vi "Y_AxisMotorControlSetupAndHome.vi"() -> ()   [LabVIEW 2020]
uses:
  C:/Program Files/National Instruments/LabVIEW 2020/examples/Instrument IO/Serial/support/Serial - Settings.ctl
  <vilib>/Instr/_visa.llb/VISA Configure Serial Port (Instr).vi
panel:
  out "read buffer 2":string
  out "read buffer 3":string
  out "7":bool
  out "6":bool
  out "5":bool
  out "4":bool
  out "3":bool
  out "8":bool
  out "2":bool
  out "1":bool
  in  "Serial Com Port":refnum<visa-resource-name>="COM3"
  out "read buffer":string
  in  "Serial Settings":T1={"baud rate"=57600, "data bits"=8, "parity"=enum."None", "stop bits"=10, "flow control"=0} {"flow control" items=["None"=0, "XON/XOFF"=1, "RTS/CTS"=2, "DTR/DSR"=4]; "stop bits" items=["1.0"=10, "1.5"=15, "2.0"=20]; "data bits" min=5 max=8 step=1; "baud rate" items=["75"=75, "110"=110, "134"=134, "150"=150, "300"=300, "600"=600, "1200"=1200, "1800"=1800, "2400"=2400, "4800"=4800, "7200"=7200, "9600"=9600, "14400"=14400, "19200"=19200, "28800"=28800, "38400"=38400, "56000"=56000, "57600"=57600, "115200"=115200, "128000"=128000, "230400"=230400]}
  out "Status Array":bool[](array[boolean])
  out "Limit Switch Status":i32 format="%b"
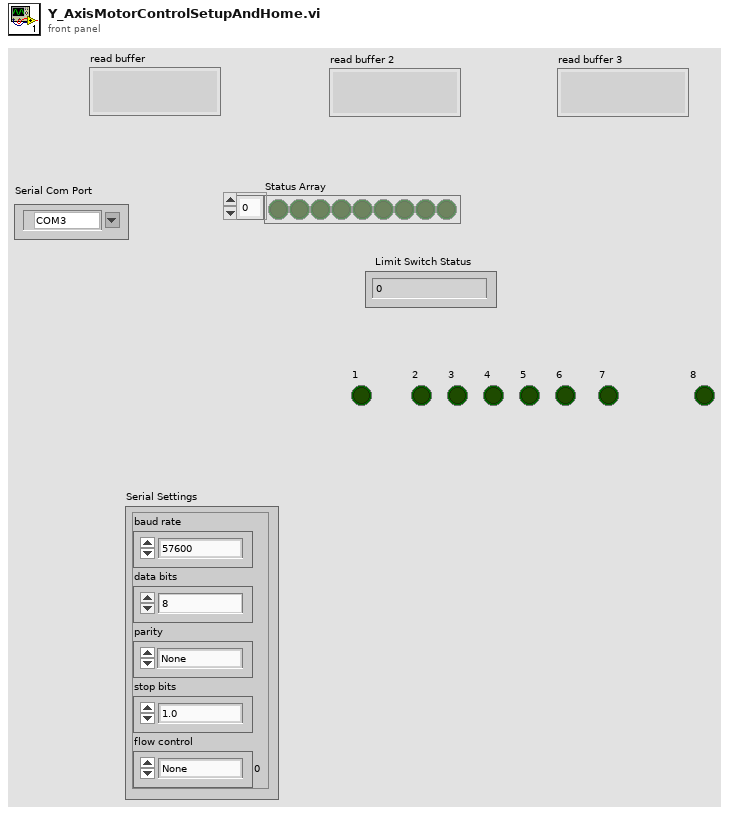
[diagram p1: front panel]
types:
  T1 = typedef "Serial - Settings.ctl" = cluster{"baud rate":u32, "data bits":u16, "parity":enum16{"None", "Odd", "Even", "Mark", "Space"}, "stop bits":u16, "flow control":u16}
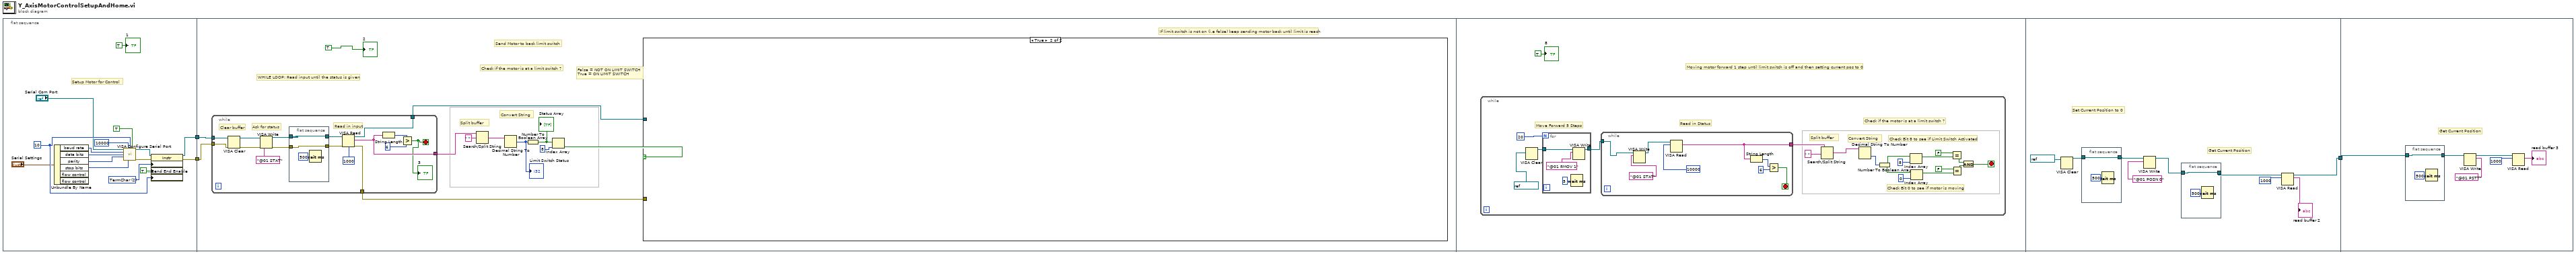
[diagram p0: block diagram]
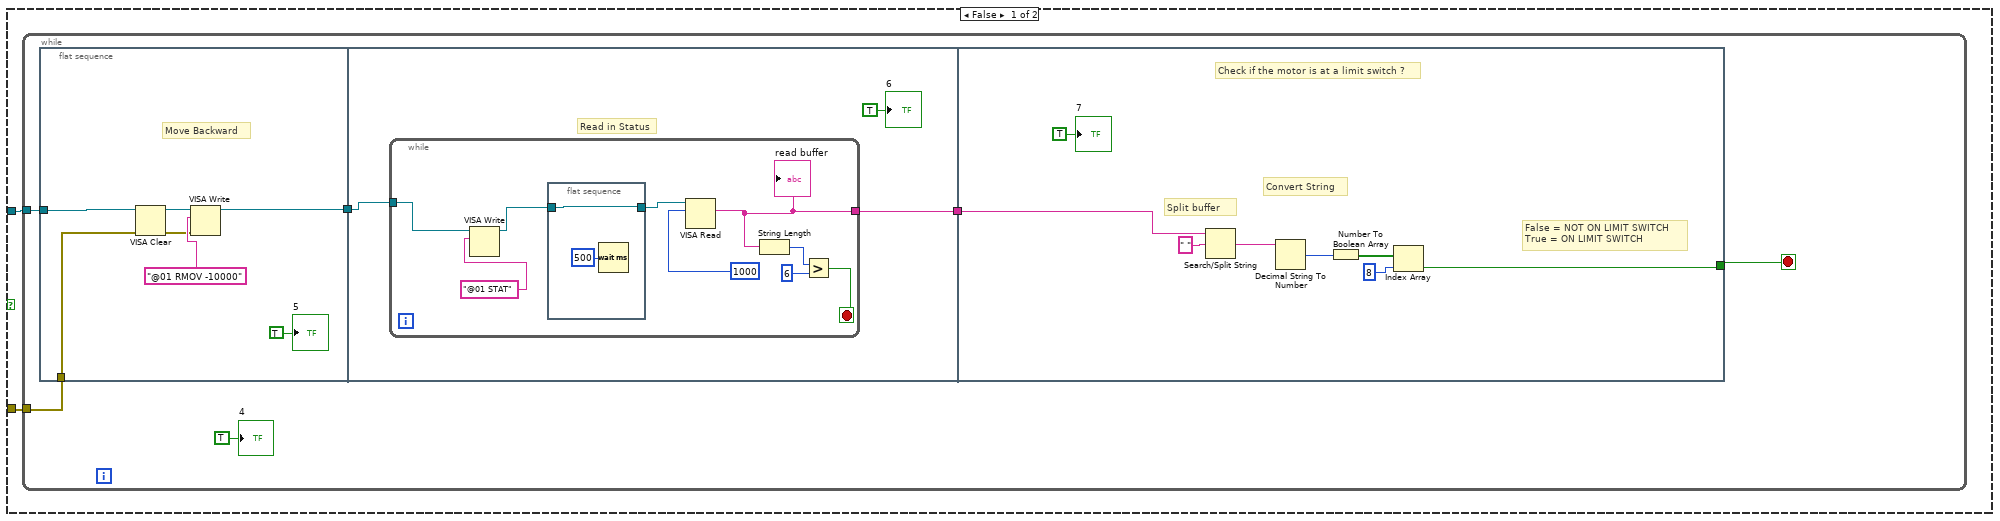
[diagram p2: hidden frame]
diagram:
  n1 = flat-sequence {
    tunnel: [w8] -> w3
    tunnel: [w5] -> w1
    tunnel: w3 -> [w25]
    tunnel: w1 -> [w22]
    tunnel: [w119] -> w2
    tunnel: w2 -> [w134]
    frame #0 {
      w9 = u8 10 ("Termination Character")
      w13 = u16 2 items=["None", "LastBit", "TermChar", "Break"] ("Serial Settings:Serial End Mode for Writes")
      # "Setup Motor for Control"
      n2 = Unbundle By Name("Serial Settings") -> ("baud rate"=w16:u32, "data bits"=w17:u16, "parity"=w18:enum16{"None", "Odd", "Even", "Mark", "Space"}, "stop bits"=w19:u16)  [unwired: 2 out]
      n3 = call-poly "VISA Configure Serial Port"("VISA resource name"="Serial Com Port", "timeout (10sec)"=u32 10000, "termination char\n(0xA = '\\n' = LF)"=w9, "Enable Termination\nChar (T)"=TRUE ("End Read on Termination Character?"), "baud rate (9600)"=w16, "data bits (8)"=w17, "parity (0:none)"=w18, "stop bits (10: 1 bit)"=w19) -> ("VISA resource name out"=w15:refnum<visa-resource-name>, "error out"=w14:errorcluster)  [unwired: 2 in, 4 out]
      n4 = property class="Instr"(reference=w15, error in=w14, "Serial Settings:End Mode for Writes"=w13, "Message Based Settings:Send End Enable"=TRUE, "Message Based Settings:Termination Character"=w9) -> (reference out=w8:refnum<visa-resource-name>, error out=w5:errorcluster)
      "1" <- TRUE ("1")
    }
    frame #1 {
      # "If limit switch is not on (i.e false) keep sending motor back until limit is reach"
      # "Send Motor to back limit switch"
      # "False = NOT ON LIMIT SWITCH \nTrue = ON LIMIT SWITCH"
      # "WHILE LOOP: Read input until the status is given"
      # "Check if the motor is at a limit switch ?"
      # "Convert String"
      # "Split buffer"
      n5 = while {
        tunnel: [w83] -> w27
        tunnel: w25 -> [w79]
        tunnel: [w75] -> w23
        tunnel: w22 -> [w74]
        tunnel: [w70] -> w21
        stop <- w69 stop-if-true
        # "Clear buffer"
        # "Ask for status"
        # "Read in input"
        n6 = VISA Clear(VISA resource name=w79, error in (no error)=w74) -> (VISA resource name out=w78:refnum<visa-resource-name>, error out=w73:errorcluster)
        n7 = VISA Write(VISA resource name=w78, write buffer="@01 STAT" ("Command 2"), error in (no error)=w73) -> (VISA resource name out=w77:refnum<visa-resource-name>, error out=w72:errorcluster)  [unwired: 1 out]
        n8 = flat-sequence {
          tunnel: w77 -> [w86]
          tunnel: [w86] -> w76
          tunnel: [w85] -> w71
          tunnel: w72 -> [w85]
          frame #0 {
            n9 = Wait (ms)(milliseconds to wait=u32 500) -> ()  [unwired: 1 out]
          }
        }
        n10 = VISA Read(VISA resource name=w76, byte count=u32 1000 ("Read Word Length Count?"), error in (no error)=w71) -> (VISA resource name out=w75:refnum<visa-resource-name>, read buffer=w83:string, error out=w70:errorcluster)  [unwired: 1 out]
        n11 = String Length(string=w83) -> (length=w82:i32)
        n12 = Greater?(x=w82, y=6) -> (0:w69:bool)
        "3" <- w69
      }
      n13 = Search/Split String(string=w27, search string/char (-)=" ") -> (match + rest of string=w30:string)  [unwired: 1 in, 2 out]
      n14 = Decimal String To Number(string=w30) -> (number=w26:i32)  [unwired: 2 in, 1 out]
      "Limit Switch Status" <- w26
      n15 = Number To Boolean Array(number=w26) -> (Boolean array=w31:bool[])
      "Status Array" <- w31
      n16 = Index Array(array=w31, index=8) -> (element=w24:bool)
      n17 = case shown="True" w24 {
        tunnel: w23 -> [w33 _]
        tunnel: w21 -> [w32 _]
        frame False {
          n18 = while {
            tunnel: w33 -> [w36]
            tunnel: w32 -> [w35]
            stop <- w38 stop-if-true
            n19 = flat-sequence {
              tunnel: [w44] -> w39
              tunnel: w36 -> [w43]
              tunnel: w35 -> [w42]
              tunnel: w39 -> [w49]
              tunnel: [w48] -> w37
              tunnel: [w64] -> w38
              tunnel: w37 -> [w63]
              frame #0 {
                # "Move Backward"
                n20 = VISA Clear(VISA resource name=w43, error in (no error)=w42) -> (VISA resource name out=w46:refnum<visa-resource-name>, error out=w41:errorcluster)
                n21 = VISA Write(VISA resource name=w46, write buffer="@01 RMOV -10000" ("Command 2"), error in (no error)=w41) -> (VISA resource name out=w44:refnum<visa-resource-name>)  [unwired: 2 out]
                "5" <- TRUE ("2 4")
              }
              frame #1 {
                # "Read in Status"
                n22 = while {
                  tunnel: [w55] -> w48
                  tunnel: w49 -> [w50]
                  stop <- w54 stop-if-true
                  n23 = VISA Write(VISA resource name=w50, write buffer="@01 STAT" ("Command 2")) -> (VISA resource name out=w51:refnum<visa-resource-name>)  [unwired: 1 in, 2 out]
                  n24 = flat-sequence {
                    tunnel: w51 -> [w59]
                    tunnel: [w59] -> w52
                    frame #0 {
                      n25 = Wait (ms)(milliseconds to wait=u32 500) -> ()  [unwired: 1 out]
                    }
                  }
                  n26 = VISA Read(VISA resource name=w52, byte count=u32 1000 ("Read Word Length Count?")) -> (read buffer=w55:string)  [unwired: 1 in, 3 out]
                  "read buffer" <- w55
                  n27 = String Length(string=w55) -> (length=w57:i32)
                  n28 = Greater?(x=w57, y=6) -> (0:w54:bool)
                }
                "6" <- TRUE ("6")
              }
              frame #2 {
                # "False = NOT ON LIMIT SWITCH \nTrue = ON LIMIT SWITCH"
                # "Check if the motor is at a limit switch ?"
                # "Convert String"
                # "Split buffer"
                n29 = Search/Split String(string=w63, search string/char (-)=" ") -> (match + rest of string=w67:string)  [unwired: 1 in, 2 out]
                n30 = Decimal String To Number(string=w67) -> (number=w62:i32)  [unwired: 2 in, 1 out]
                n31 = Number To Boolean Array(number=w62) -> (Boolean array=w68:bool[])
                n32 = Index Array(array=w68, index=8) -> (element=w64:bool)
                "7" <- TRUE ("7")
              }
            }
            "4" <- TRUE ("2 3")
          }
        }
        frame True {
        }
      }
      "2" <- TRUE ("1")
    }
    frame #2 {
      # "Moving motor forward 1 step until limit switch is off and then setting current pos to 0"
      n33 = while {
        stop <- w99 stop-if-true
        # "Check Bit 0 to see if motor is moving"
        # "Check if the motor is at a limit switch ?"
        # "Read in Status"
        # "Move Forward 5 Steps"
        # "Check Bit 8 to see if Limit Switch Activated"
        # "Convert String"
        # "Split buffer"
        n34 = VISA Clear(VISA resource name=refnum<visa-resource-name> "COM3" ("VISA resource name out")) -> (VISA resource name out=w90:refnum<visa-resource-name>)  [unwired: 1 in, 1 out]
        n35 = for {
          N: 20 -> [_]
          tunnel: [w109] -> w92
          tunnel: w90 -> [w107]
          n36 = Wait (ms)(milliseconds to wait=u32 5) -> ()  [unwired: 1 out]
          n37 = VISA Write(VISA resource name=w107, write buffer="@01 RMOV 1" ("Command 2")) -> (VISA resource name out=w109:refnum<visa-resource-name>)  [unwired: 1 in, 2 out]
        }
        n38 = while {
          tunnel: [w115] -> w102
          tunnel: w92 -> [w111]
          stop <- w114 stop-if-true
          n39 = VISA Write(VISA resource name=w111, write buffer="@01 STAT" ("Command 2")) -> (VISA resource name out=w113:refnum<visa-resource-name>)  [unwired: 1 in, 2 out]
          n40 = VISA Read(VISA resource name=w113, byte count=u32 10000 ("Read Word Length Count?")) -> (read buffer=w115:string)  [unwired: 1 in, 3 out]
          n41 = String Length(string=w115) -> (length=w117:i32)
          n42 = Greater?(x=w117, y=6) -> (0:w114:bool)
        }
        n43 = Search/Split String(string=w102, search string/char (-)=" ") -> (match + rest of string=w105:string)  [unwired: 1 in, 2 out]
        n44 = Decimal String To Number(string=w105) -> (number=w106:i32)  [unwired: 2 in, 1 out]
        n45 = Number To Boolean Array(number=w106) -> (Boolean array=w94:bool[])
        n46 = Index Array(array=w94, index=8) -> (element=w101:bool)
        n47 = Index Array(array=w94, index=0) -> (element=w96:bool)
        n48 = Equal?(x=FALSE, y=w101) -> (x = y?=w98:bool)
        n49 = Equal?(x=FALSE, y=w96) -> (x = y?=w93:bool)
        n50 = And(x=w98, y=w93) -> (x .and. y?=w99:bool)
      }
      "8" <- TRUE ("3")
    }
    frame #3 {
      # "Get Current Position"
      # "Set Current Position to 0"
      n51 = VISA Clear(VISA resource name=refnum<visa-resource-name> "COM3" ("VISA resource name out")) -> (VISA resource name out=w125:refnum<visa-resource-name>)  [unwired: 1 in, 1 out]
      n52 = flat-sequence {
        tunnel: w125 -> [w130]
        tunnel: [w130] -> w124
        frame #0 {
          n53 = Wait (ms)(milliseconds to wait=u32 500) -> ()  [unwired: 1 out]
        }
      }
      n54 = VISA Write(VISA resource name=w124, write buffer="@01 POSN 0" ("Command 2")) -> (VISA resource name out=w121:refnum<visa-resource-name>)  [unwired: 1 in, 2 out]
      n55 = flat-sequence {
        tunnel: w121 -> [w128]
        tunnel: [w128] -> w120
        frame #0 {
          n56 = Wait (ms)(milliseconds to wait=u32 500) -> ()  [unwired: 1 out]
        }
      }
      n57 = VISA Read(VISA resource name=w120, byte count=u32 1000 ("Read Word Length Count?")) -> (VISA resource name out=w119:refnum<visa-resource-name>, read buffer=→"read buffer 2":string)  [unwired: 1 in, 2 out]
    }
    frame #4 {
      # "Get Current Position"
      n58 = flat-sequence {
        tunnel: w134 -> [w138]
        tunnel: [w138] -> w133
        frame #0 {
          n59 = Wait (ms)(milliseconds to wait=u32 500) -> ()  [unwired: 1 out]
        }
      }
      n60 = VISA Write(VISA resource name=w133, write buffer="@01 PSTT" ("Command 2")) -> (VISA resource name out=w137:refnum<visa-resource-name>)  [unwired: 1 in, 2 out]
      n61 = VISA Read(VISA resource name=w137, byte count=u32 1000 ("Read Word Length Count?")) -> (read buffer=→"read buffer 3":string)  [unwired: 1 in, 3 out]
    }
  }
